vi "Get Active Guidance.vi"(8 "error in (no error)":errorcluster, 11 "Vessel in":refnum<class "Vessel.lvclass">) -> (0 "error out":errorcluster, 2 "Guidance Out":refnum<class "Guidance.lvclass">, 3 "Vessel out":refnum<class "Vessel.lvclass">)   [LabVIEW 2014, in "Vessel.lvclass"]
uses:
  Vessel.lvclass
  Guidance/Guidance.lvclass
  Vessel.lvclass/Vessel.ctl
  Supervisor/Supervisor.lvclass
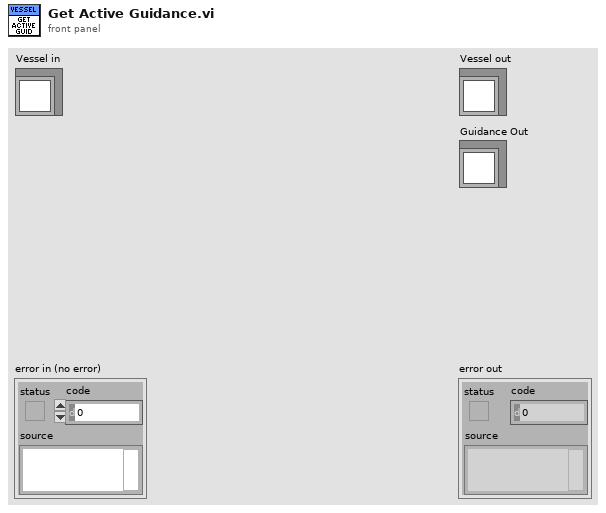
[diagram p1: front panel]
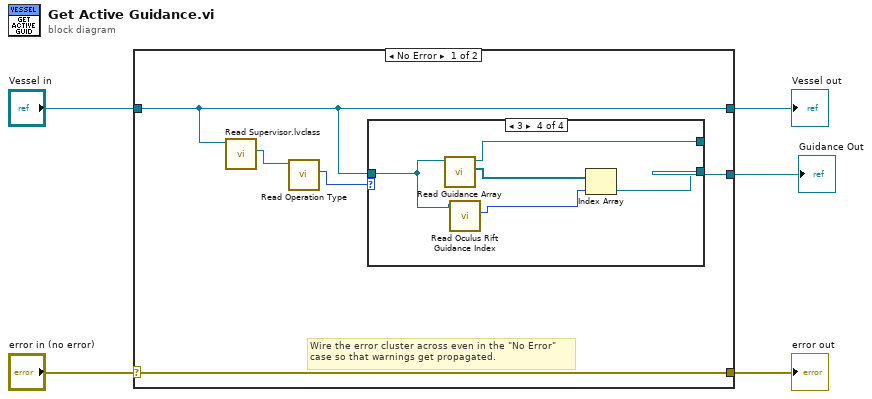
[diagram p0: block diagram]
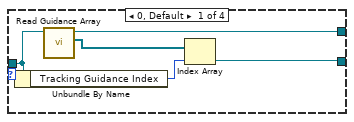
[diagram p2: hidden frame]
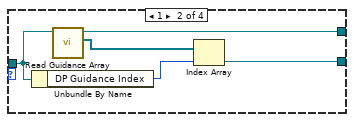
[diagram p3: hidden frame]
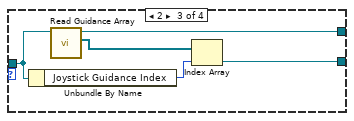
[diagram p4: hidden frame]
diagram:
  n1 = case shown="No Error" "error in (no error)" {
    selector: "error in (no error)" -> [w10 w32]
    tunnel: [w10 w32] -> w4
    tunnel: [w8 w31] -> w2
    tunnel: "Vessel in" -> [w8 w31]
    tunnel: [w6 _] -> w1
    frame No Error {
      # "Wire the error cluster across even in the \"No Error\"\ncase so that warnings get propagated."
      n2 = call "Read Supervisor.lvclass.vi"("Vessel in"=w8) -> ("Supervisor.lvclass"=w9:refnum<class "Supervisor.lvclass">)  [unwired: 8 in, 2 out]
      n3 = call-dynamic "Read Operation Type.vi"("Supervisor in"=w9) -> ("Operation Type"=w7:u16)  [unwired: 8 in, 2 out]
      n4 = case shown="3" w7 {
        tunnel: w8 -> [w15 w20 w25 w27]
        tunnel: [w12 w17 w23 w29] -> _
        tunnel: [w11 w16 w21 w28] -> w6
        frame 0, Default {
          n5 = Unbundle By Name(w15) -> ("Tracking Guidance Index"=w14:i32)
          n6 = call "Read Guidance Array.vi"("Vessel in"=w15) -> ("Guidance Array"=w13:refnum<class "Guidance.lvclass">[], "Vessel out"=w12:refnum<class "Vessel.lvclass">)  [unwired: 8 in, 1 out]
          n7 = Index Array(array=w13, index=w14) -> (element=w11:refnum<class "Guidance.lvclass">)
        }
        frame 1 {
          n8 = Unbundle By Name(w20) -> ("DP Guidance Index"=w18:i32)
          n9 = call "Read Guidance Array.vi"("Vessel in"=w20) -> ("Guidance Array"=w19:refnum<class "Guidance.lvclass">[], "Vessel out"=w17:refnum<class "Vessel.lvclass">)  [unwired: 8 in, 1 out]
          n10 = Index Array(array=w19, index=w18) -> (element=w16:refnum<class "Guidance.lvclass">)
        }
        frame 2 {
          n11 = Unbundle By Name(w25) -> ("Joystick Guidance Index"=w22:i32)
          n12 = call "Read Guidance Array.vi"("Vessel in"=w25) -> ("Guidance Array"=w24:refnum<class "Guidance.lvclass">[], "Vessel out"=w23:refnum<class "Vessel.lvclass">)  [unwired: 8 in, 1 out]
          n13 = Index Array(array=w24, index=w22) -> (element=w21:refnum<class "Guidance.lvclass">)
        }
        frame 3 {
          n14 = call "Read Guidance Array.vi"("Vessel in"=w27) -> ("Guidance Array"=w30:refnum<class "Guidance.lvclass">[], "Vessel out"=w29:refnum<class "Vessel.lvclass">)  [unwired: 8 in, 1 out]
          n15 = call-dynamic "Read Oculus Rift Guidance Index.vi"("Vessel in"=w27) -> ("Oculus Rift Guidance Index"=w26:i32)  [unwired: 8 in, 2 out]
          n16 = Index Array(array=w30, index=w26) -> (element=w28:refnum<class "Guidance.lvclass">)
        }
      }
    }
    frame Error {
    }
  }
  "error out" <- w4
  "Vessel out" <- w2
  "Guidance Out" <- w1
